vi "Impedance Model v2.vi"(8 "Theta_d":dbl, 9 "K":dbl, 11 "Sensors":T1) -> (2 "Tau_ref":dbl)   [LabVIEW 2018]
uses:
  Sensor Data.ctl
panel:
  out "Theta":dbl(graph)=0.4035824604253701
  out "ILC Theta":dbl(graph)=0.4035824604253701
  out "Torque Reference":dbl(graph)=0.4035824604253701
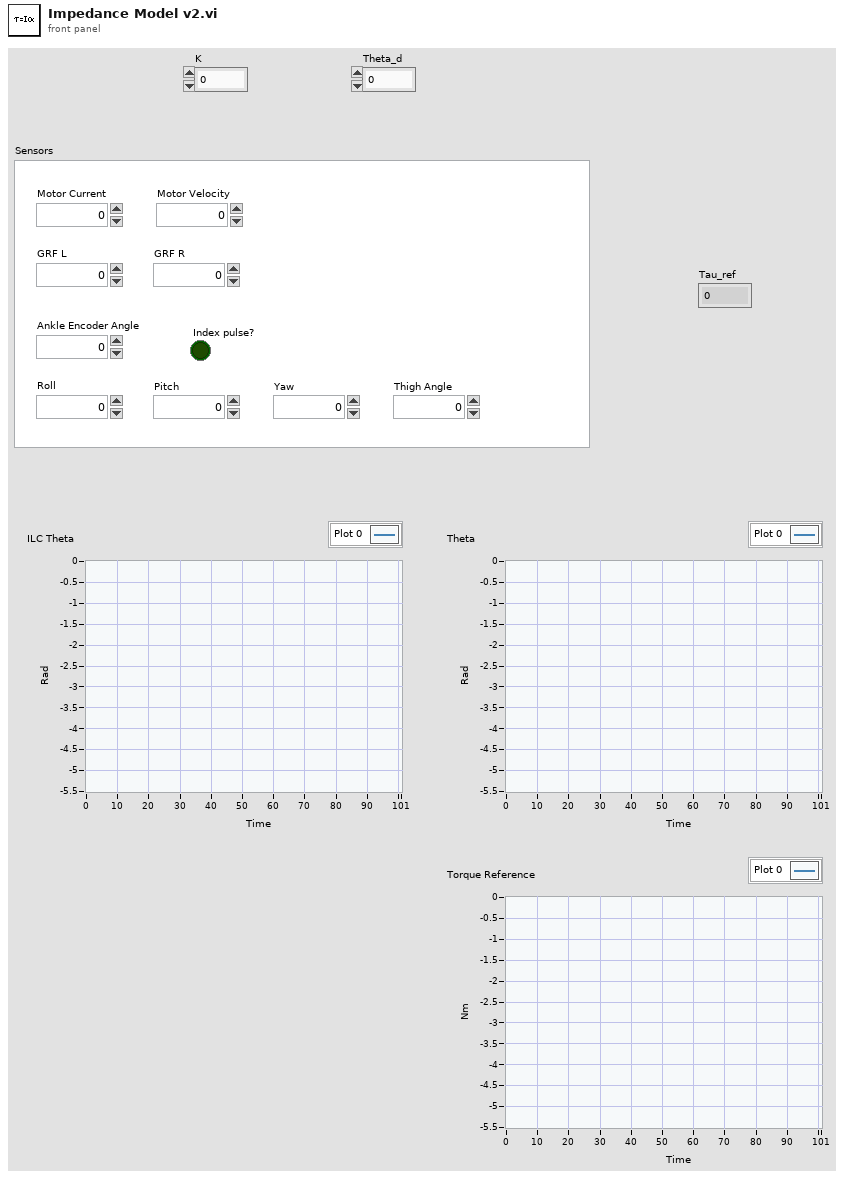
[diagram p1: front panel]
types:
  T1 = typedef "Sensor Data.ctl" = cluster{"Motor Current":dbl, "Motor Velocity":dbl, "Ankle Encoder Angle":dbl, "GRF L":dbl, "GRF R":dbl, "Index pulse?":bool, "Roll":dbl, "Pitch":dbl, "Yaw":dbl, "Thigh Angle":dbl}
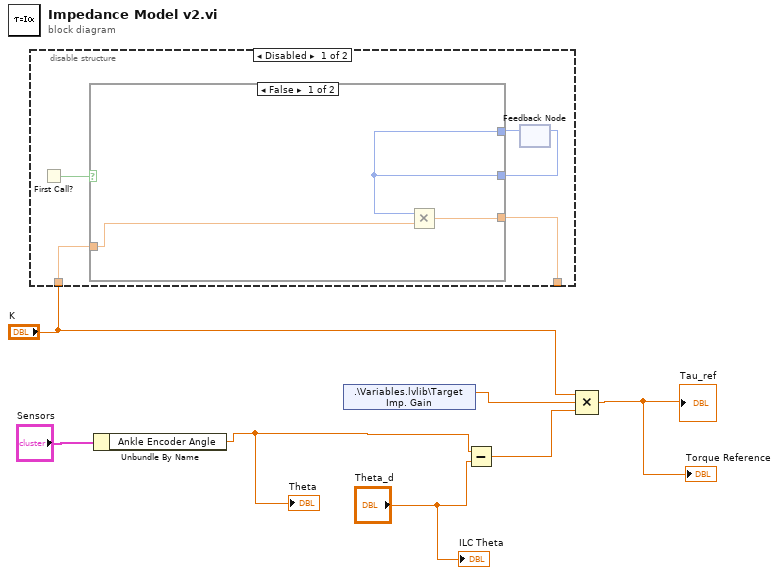
[diagram p0: block diagram]
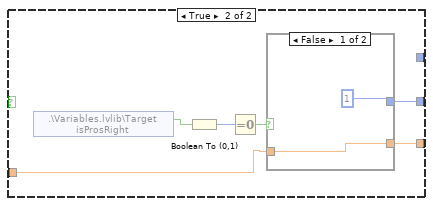
[diagram p2: hidden frame]
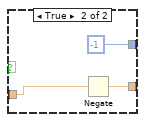
[diagram p3: hidden frame]
diagram:
  n1 = disable-structure shown="Disabled" {
    disable-tunnel: "K" -> [w11 _]
    disable-tunnel: [w10 _] -> _
    frame Disabled {
      n2 = First Call?() -> (First Call?: T/F=w12:bool)
      n3 = feedback #1() -> (w9:i32)  [unwired: 1 in]
      n4 = case shown="False" w12 {
        tunnel: w11 -> [w14 w18]
        tunnel: [w15 w17] -> w10
        tunnel: w9 -> [w13 _]
        tunnel: [w13 w16] -> w8
        frame False {
          n5 = Multiply(x=w13, y=w14) -> (x*y=w15:dbl)
        }
        frame True {
          n6 = shared-variable ".\\Variables.lvlib\\Target isProsRight"() -> (w21:bool)  [unwired: 1 in, 1 out]
          n7 = Boolean To (0,1)(Boolean=w21) -> (0, 1=w20:i16)
          n8 = Equal To 0?(x=w20) -> (x = 0?=w19:bool)
          n9 = case shown="False" w19 {
            tunnel: w18 -> [w23 w26]
            tunnel: [w23 w25] -> w17
            tunnel: [1 -1] -> w16
            frame False {
            }
            frame True {
              n10 = Negate(x=w26) -> (-x=w25:dbl)
            }
          }
        }
      }
      n11 = feedback-in #1(w8) -> ()
    }
    frame Enabled {
    }
  }
  n12 = Unbundle By Name("Sensors") -> ("Ankle Encoder Angle"=w5:dbl)
  "Theta" <- w5
  n13 = shared-variable ".\\Variables.lvlib\\Target Imp. Gain"() -> (w2:dbl)  [unwired: 1 in, 1 out]
  n14 = Subtract(x=w5, y="Theta_d") -> (x-y=w3:dbl)
  n15 = Compound Arithmetic op=MULTIPLY("K", w2, w3) -> (→"Tau_ref" →"Torque Reference":dbl)
  "ILC Theta" <- "Theta_d"
